vi "Helper SubVI - Debugging Disabled.vi"(10 "Numeric In":dbl) -> (2 "Numeric Out":dbl)   [LabVIEW 2023]
doc: "This VI has normal priority and debugging disabled. Disabling debugging has a small performance impact."
panel:
  # "This VI has debugging disabled in its execution properties."
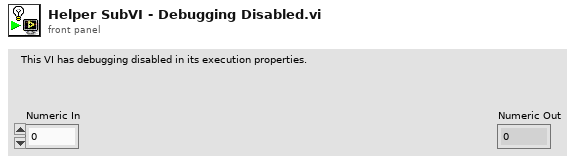
[diagram p1: front panel]
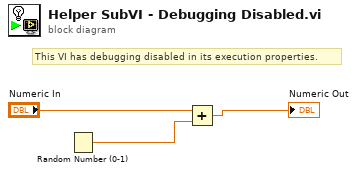
[diagram p0: block diagram]
diagram:
  # "This VI has debugging disabled in its execution properties."
  n1 = Random Number (0-1)() -> (number: 0 to 1=w1:dbl)
  n2 = Add(x="Numeric In", y=w1) -> (x+y=→"Numeric Out":dbl)
